vi "pp2_sessList_isValid.vi"(0 "Trial Types In":T1[](array[typedef])=[{"Trial Type Number"=1, "Trial Type"=enum."GO", "Trial Weight"=1, "Shock (mA)"=-1.0, "Duration (ms)"=250.0, "Sound Type"=enum."04 FM Sweep", "Stim P1"=2000.0, "Stim P2"=4000.0, "Stim P3"=0.0, "Stim P4"=0.0}, {"Trial Type Number"=2, "Trial Type"=enum."NOGO", "Trial Weight"=1, "Shock (mA)"=-1.0, "Duration (ms)"=250.0, "Sound Type"=enum."04 FM Sweep", "Stim P1"=4000.0, "Stim P2"=2000.0, "Stim P3"=0.0, "Stim P4"=0.0}, {"Trial Type Number"=3, "Trial Type"=enum."TEST", "Trial Weight"=0, "Shock (mA)"=0.0, "Duration (ms)"=0.0, "Sound Type"=enum."00 NULL", "Stim P1"=0.0, "Stim P2"=0.0, "Stim P3"=0.0, "Stim P4"=0.0}, {"Trial Type Number"=4, "Trial Type"=enum."NOGO", "Trial Weight"=0, "Shock (mA)"=0.0, "Duration (ms)"=0.0, "Sound Type"=enum."00 NULL", "Stim P1"=0.0, "Stim P2"=0.0, "Stim P3"=0.0, "Stim P4"=0.0}] {"Shock (mA)" min=-1.0 max=5.0; "Trial Weight" step=1; "Duration (ms)" min=0.0 max=1.0; "Trial Type Number" min=1 max=256 step=1}, 5 "Total Trials":i32=60 min=2 step=2, 9 "Session List":i32[](array[numeric])=[1, 1, 1, 2, 2, 1, 2, 1, 1, 2, 2, 2, 1, 1, 2, 2, 1, 2, 1, 1, 2, 2, 1, 2, 1, 1, 1, 2, 1, 2, 1, 2, 1, 2, 2, 1, 2, 1, 2, 1, 2, 2, 1, 2, 2, 1, 2, 1, 2, 2, 1, 1, 2, 1, 2, 2, 1, 2, 1, 1], 13 "Trial Replication Factor":i32) -> (4 "Session List Valid?":bool=TRUE)   [LabVIEW 2013]
uses:
  pp2_CTL_Trial.ctl
  pp2_CTL_TrialType.ctl
  labolabo2/waveforms/WFTypes.ctl
  labolabo2/array/impl/ArrayRemove_I.vi
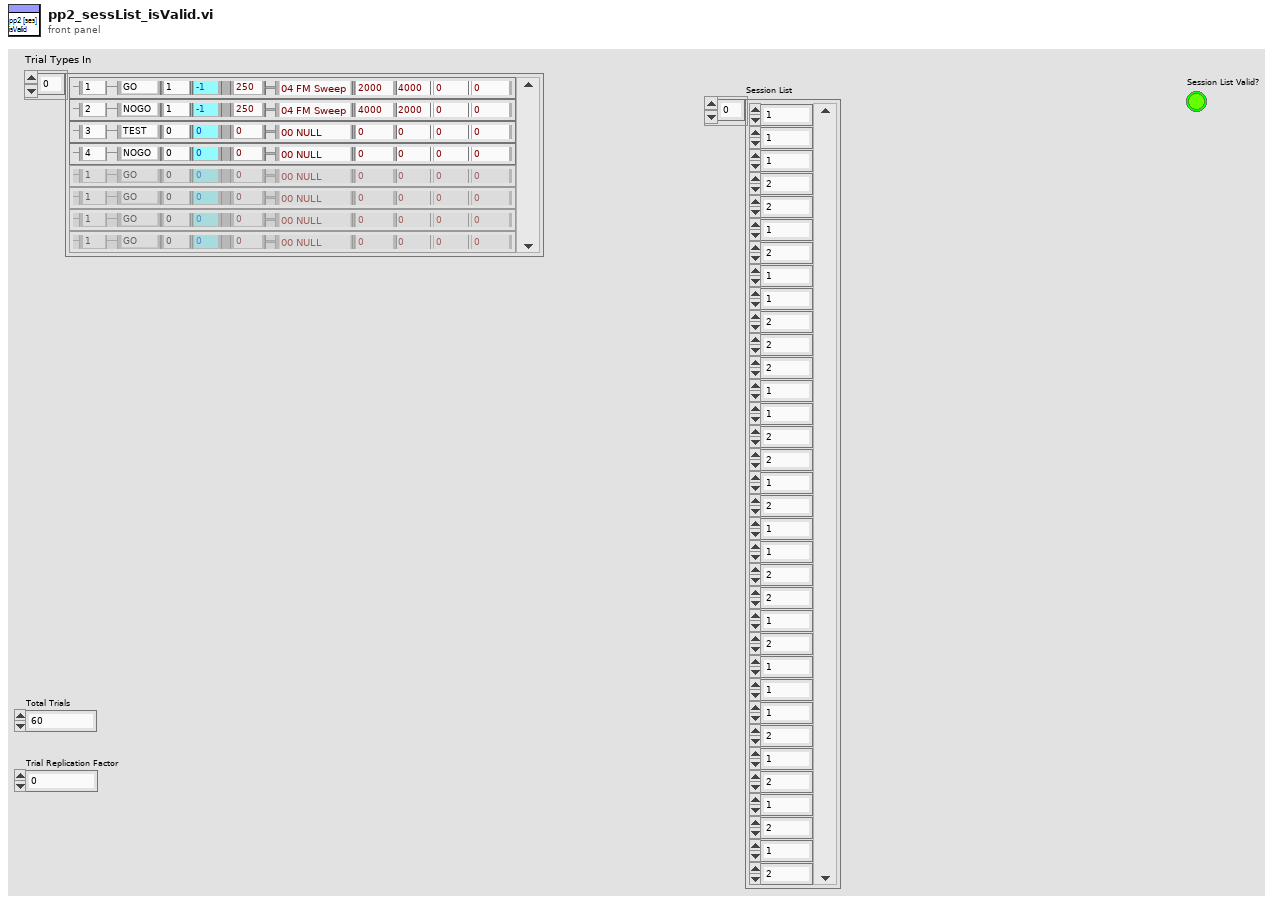
[diagram p1: front panel]
types:
  T1 = typedef "pp2_CTL_Trial.ctl" = cluster{"Trial Type Number":i16, "Trial Type":T2, "Trial Weight":u32, "Shock (mA)":dbl, "Duration (ms)":dbl, "Sound Type":T3, "Stim P1":dbl, "Stim P2":dbl, "Stim P3":dbl, "Stim P4":dbl}
  T2 = typedef "pp2_CTL_TrialType.ctl" = enum16{"OFF", "GO", "NOGO", "TEST"}
  T3 = typedef "WFTypes.ctl" = enum16{"00 NULL", "01 DC", "02 Noise", "03 Pure Tone", "04 FM Sweep"}
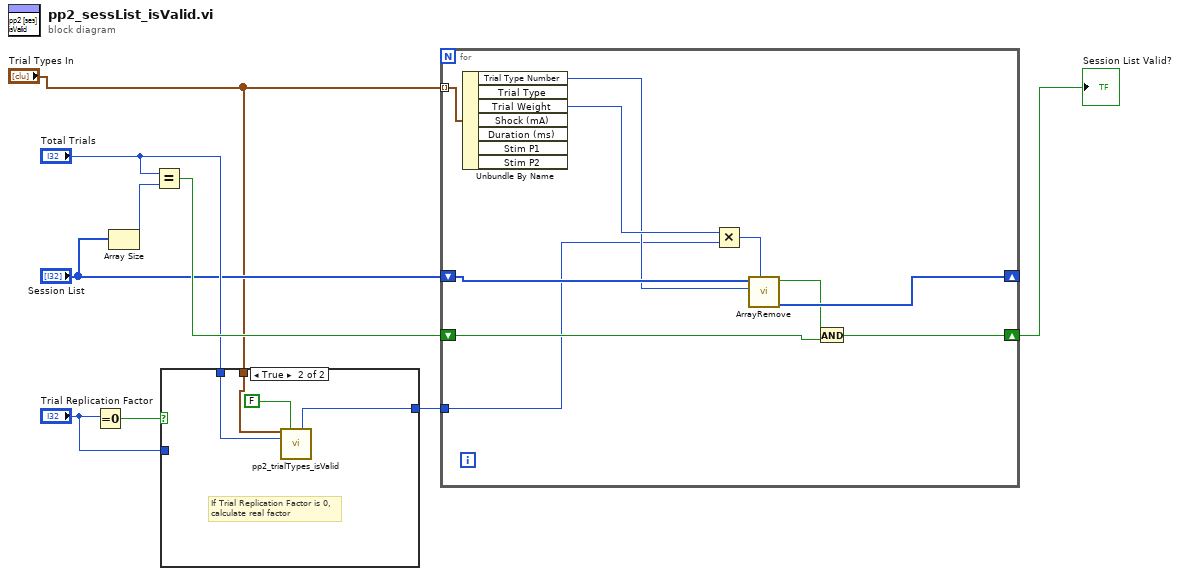
[diagram p0: block diagram]
diagram:
  n1 = Equal To 0?(x="Trial Replication Factor") -> (x = 0?=w6:bool)
  n2 = Array Size(array="Session List") -> (size(s)=w9:i32)
  n3 = Equal?(x="Total Trials", y=w9) -> (x = y?=w8:bool)
  n4 = case shown="True" w6 {
    tunnel: "Trial Replication Factor" -> [w10 _]
    tunnel: [w10 w14] -> w3
    tunnel: "Trial Types In" -> [_ w11]
    tunnel: "Total Trials" -> [_ w13]
    frame False {
    }
    frame True {
      # "If Trial Replication Factor is 0,\ncalculate real factor"
      n5 = call "pp2_trialTypes_isValid.vi"("Trial Types In"=w11, "Throw Error"=FALSE, "Total Trials"=w13) -> ("Trial Replication Factor"=w14:i32)  [unwired: 7 in, 5 out]
    }
  }
  n6 = for {
    tunnel: "Trial Types In" -> [w15] mode=indexing
    shift-right: [w17] -> w7
    shift-left: w8 -> [w21]
    tunnel: w3 -> [w16]
    shift-right: [w23] -> _
    shift-left: "Session List" -> [w24]
    n7 = Unbundle By Name(w15) -> ("Trial Type Number"=w18:i16, "Trial Weight"=w20:u32)  [unwired: 5 out]
    n8 = Multiply(x=w20, y=w16) -> (x*y=w19:u32)
    n9 = call-poly "ArrayRemove.vi"("How many to remove"=w19, "To Remove"=w18, "1D Array In"=w24) -> ("1D Array Out"=w23:i32[], "Removed All"=w22:bool)  [unwired: 7 in]
    n10 = And(x=w22, y=w21) -> (x .and. y?=w17:bool)
  }
  "Session List Valid?" <- w7
